vi "Set Mode.vi"(0 "comm interface in":refnum<class "Pixy Com.lvclass">, 5 "mode":u8 format="%.0x", 11 "error in":errorcluster) -> (4 "comm interface out":refnum<class "Pixy Com.lvclass">, 15 "error out":errorcluster)   [LabVIEW 2018, in "Pixy2.lvlib"]
doc: "Configures Line Tracking algorithm parameters. OR modes together if you'd like to set more than one.\n\nModes:\n0x01 - LINE_MODE_TURN_DELAYED\n0x02 - LINE_MODE_MANUAL_SELECT_VECTOR\n0x80 - LINE_MODE_WHITE_LINE"
uses:
  Pixy2.lvlib
  Interface/Pixy Com.lvclass
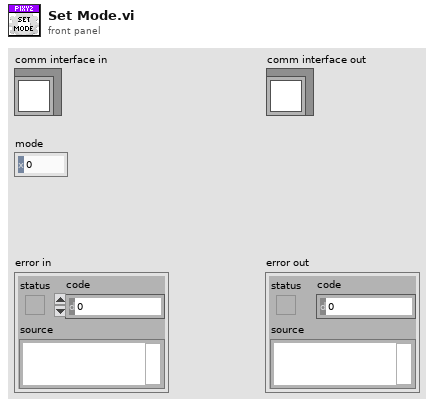
[diagram p1: front panel]
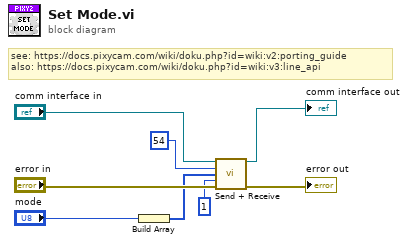
[diagram p0: block diagram]
diagram:
  # "see: https://docs.pixycam.com/wiki/doku.php?id=wiki:v2:porting_guide\nalso: https://docs.pixycam.com/wiki/doku.php?id=wiki:v3:line_api"
  n1 = Build Array("mode") -> (w1:u8[])
  n2 = call "Send + Receive.vi"("comm interface in"="comm interface in", "type"=u8 54, "payload"=w1, "expected response"=u8 1 ("expected type"), "error in"="error in") -> ("comm interface out"=→"comm interface out":refnum<class "Pixy Com.lvclass">, "error out"=→"error out":errorcluster)  [unwired: 8 in, 1 out]
